vi "FFT_test.vi"(10 "Array - Numeric 2":i32[](array[numeric]), 11 "Array - Numeric":i32[](array[numeric])) -> (3 "Magnitude":dbl[](array[numeric]))   [LabVIEW 2014]
uses:
  <vilib>/Analysis/2dsp.llb/Real FFT.vi
  <vilib>/Analysis/NI_AALPro.lvlib
  <vilib>/ptbypt/NI_PtbyPt.lvlib
panel:
  out "Array length":i32
  out "Phase":dbl[](array[numeric])
  out "Array - Numeric 3":i32[](array[numeric])
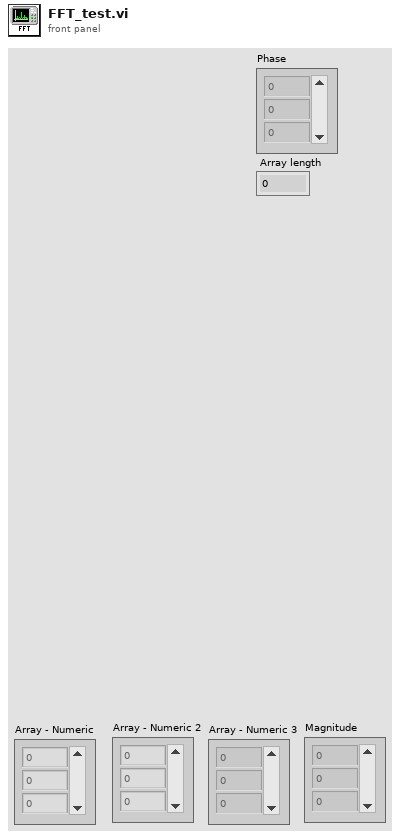
[diagram p1: front panel]
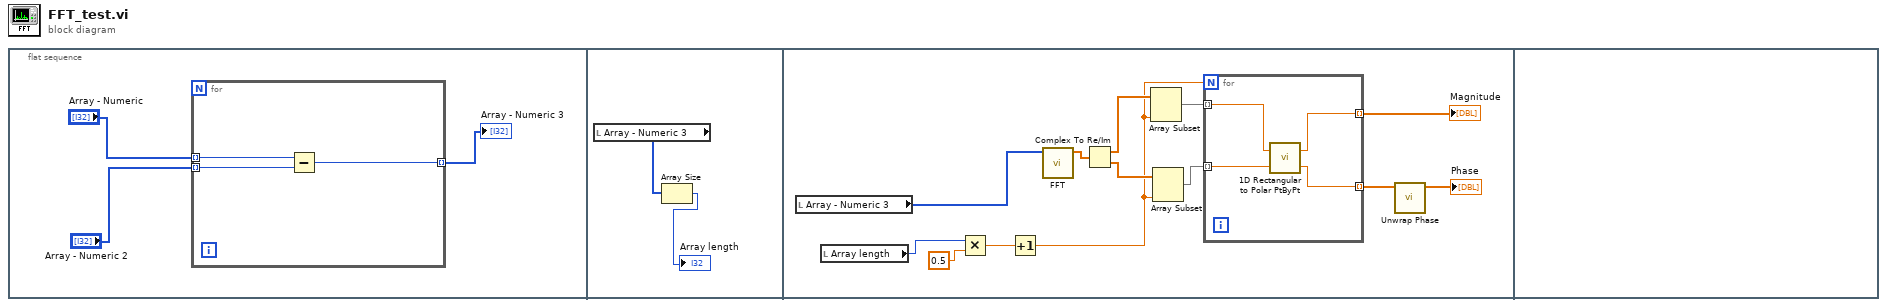
[diagram p0: block diagram]
diagram:
  n1 = flat-sequence {
    frame #0 {
      n2 = for {
        tunnel: "Array - Numeric" -> [w6] mode=indexing
        tunnel: "Array - Numeric 2" -> [w5] mode=indexing
        tunnel: [w4] -> w1 mode=indexing
        n3 = Subtract(x=w6, y=w5) -> (x-y=w4:i32)
      }
      "Array - Numeric 3" <- w1
    }
    frame #1 {
      n4 = local read "Array - Numeric 3"() -> (w8:i32[])
      n5 = Array Size(array=w8) -> (size(s)=→"Array length":i32)
    }
    frame #2 {
      n6 = local read "Array - Numeric 3"() -> (w20:i32[])
      n7 = local read "Array length"() -> (w19:i32)
      n8 = Multiply(x=w19, y=0.5) -> (x*y=w17:dbl)
      n9 = Increment(x=w17) -> (x+1=w14:dbl)
      n10 = call-poly <vilib>:"FFT.vi"("X"=w20) -> ("FFT {X}"=w21:cdb[])  [unwired: 9 in, 1 out]
      n11 = Complex To Re/Im(x + iy=w21) -> (x=w16:dbl[], y=w15:dbl[])
      n12 = Array Subset(array=w16, length=w14) -> (w13:dbl[])  [unwired: 1 in]
      n13 = Array Subset(array=w15, length=w14) -> (w12:dbl[])  [unwired: 1 in]
      n14 = for {
        N: w14 -> [_]
        tunnel: w13 -> [w25] mode=indexing
        tunnel: w12 -> [w24] mode=indexing
        tunnel: [w23] -> w11 mode=indexing
        tunnel: [w22] -> w10 mode=indexing
        n15 = call <vilib>:"1D Rectangular to Polar PtByPt.vi"("y"=w24, "x"=w25) -> ("phase"=w22:dbl, "magnitude"=w23:dbl)
      }
      "Magnitude" <- w11
      n16 = call <vilib>:"Unwrap Phase.vi"("Phase"=w10) -> ("Unwrapped Phase"=→"Phase":dbl[])  [unwired: 9 in, 1 out]
    }
    frame #3 {
    }
  }
